vi "CSV File.vi"(6 "Operation":enum16{"Read", "Write"}(ring), 7 "Path":path, 8 "error in":errorcluster, 10 "Write data":string[][](array[string])) -> (0 "error out":errorcluster, 2 "Pathout":path, 3 "Read Data":string[][](array[string]))   [LabVIEW 2017]
uses:
  <vilib>/Utility/file.llb/Read Delimited Spreadsheet (string).vi
  <vilib>/Utility/file.llb/Write Delimited Spreadsheet (string).vi
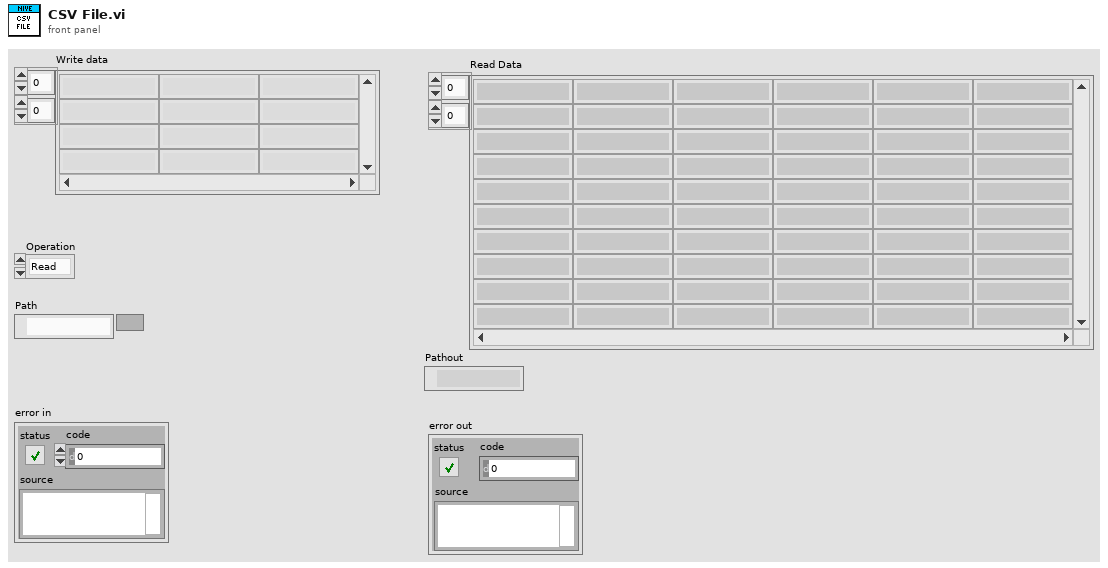
[diagram p1: front panel]
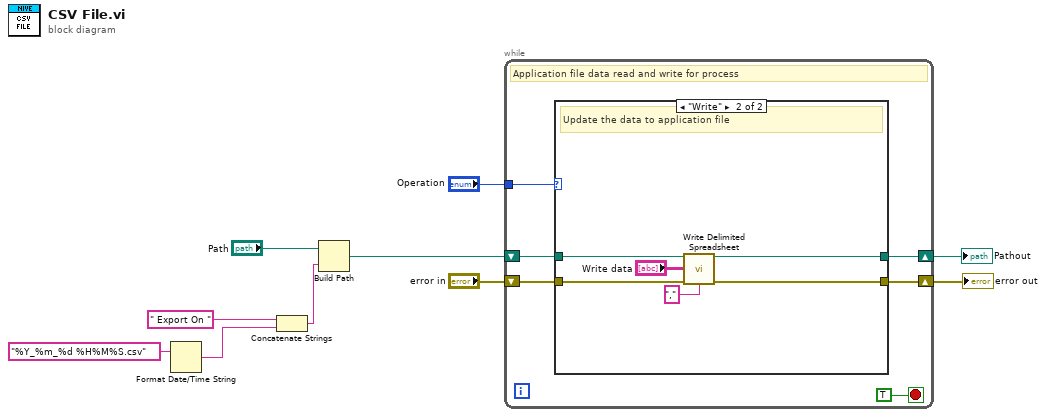
[diagram p0: block diagram]
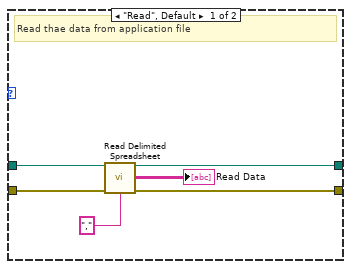
[diagram p2: hidden frame]
diagram:
  n1 = Format Date/Time String(time format string (%c)="%Y_%m_%d %H%M%S.csv") -> (date/time string=w7:string)  [unwired: 2 in]
  n2 = Concatenate Strings(" Export On ", w7) -> (w3:string)
  n3 = Build Path(base path="Path", name or relative path=w3) -> (appended path=w2:path)
  n4 = while {
    tunnel: "Operation" -> [w16]
    shift-right: [w14] -> w1
    shift-left: w2 -> [w13]
    shift-right: [w12] -> w8
    shift-left: "error in" -> [w15]
    stop <- TRUE stop-if-true
    # "Application file data read and write for process"
    n5 = case shown="\"Write\"" w16 {
      tunnel: w15 -> [w22 w28]
      tunnel: w13 -> [w21 w26]
      tunnel: [w20 w25] -> w14
      tunnel: [w19 w27] -> w12
      frame "Read", Default {
        # "Read thae data from application file"
        n6 = call-poly <vilib>:"Read Delimited Spreadsheet.vi"("file path (dialog if empty)"=w21, "error in (no error)"=w22, "delimiter (\\t)"="," ("delimiter (\\t)")) -> ("new file path (Not A Path if cancelled)"=w20:path, "all rows"=→"Read Data":string[][], "error out"=w19:errorcluster)  [unwired: 7 in, 3 out]
      }
      frame "Write" {
        # "Update the data to application file"
        n7 = call-poly <vilib>:"Write Delimited Spreadsheet.vi"("file path (dialog if empty)"=w26, "2D data"="Write data", "error in (no error)"=w28, "delimiter (\\t)"="," ("delimiter (\\t)")) -> ("new file path (Not A Path if cancelled)"=w25:path, "error out"=w27:errorcluster)  [unwired: 10 in]
      }
    }
  }
  "error out" <- w8
  "Pathout" <- w1
